vi "Check DataType with Cacher.vi"(0 "key":string, 2 "Type":T1) -> (4 "cacher":variant, 5 "match?":bool, 6 "stored type":T1, 7 "error out":errorcluster)   [LabVIEW 2017]
uses:
  <vilib>/Utility/Data Type/Type Definitions/Data Type.ctl
  <vilib>/Utility/Data Type/NI_Data Type.lvlib
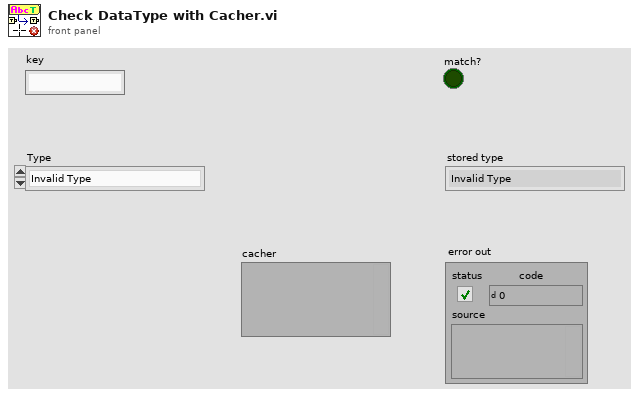
[diagram p1: front panel]
types:
  T1 = typedef "NI_Data Type.lvlib/Data Type.ctl" = enum8{"Invalid Type", "Void", "I8", "I16", "I32", "I64", "U8", "U16", "U32", "U64", "Single Float", "Double Float", "Extended Float", "Single Complex", "Double Complex", "Extended Complex", "Enum U8", "Enum U16", "Enum U32", "Enum U64", "Single Float With Unit", "Double Float With Unit", "Extended Float With Unit", "Single Complex with Unit", "Double Complex with Unit", "Extended Complex with Unit", "Boolean", "String", "Path", "Picture", "Tag", "Array", "Cluster", "Variant", "LV Variant", "Waveform", "Timestamp", "Digital Waveform", "Digital Data", "ExpressData", "Refnum", "External Data", "VI", "Poly VI", "LabVIEW Class Instance", "Fixed Point"}
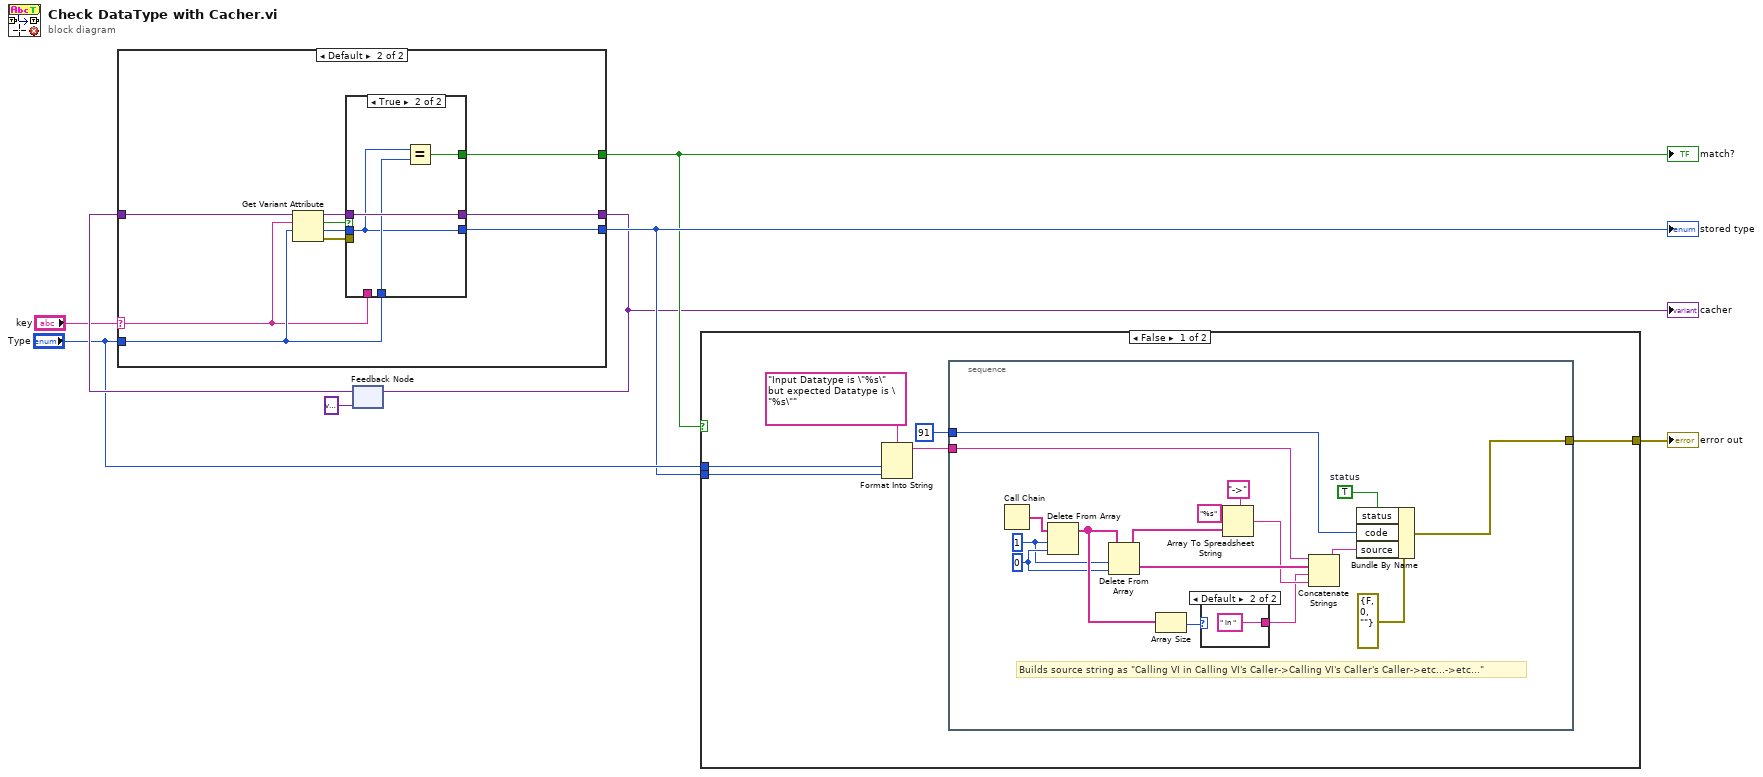
[diagram p0: block diagram]
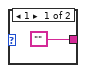
[diagram p2: hidden frame]
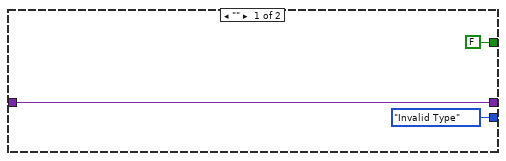
[diagram p4: hidden frame]
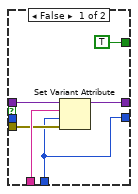
[diagram p5: hidden frame]
diagram:
  n1 = feedback #1(variant) -> (w7:variant)
  n2 = case shown="Default" "key" {
    selector: "key" -> [_ w16]
    tunnel: w7 -> [w11 w13]
    tunnel: [w11 w12] -> w1
    tunnel: "Type" -> [_ w17]
    tunnel: [FALSE w15] -> w2
    tunnel: [Data_Type."Invalid Type" ("Type") w14] -> w3
    frame "" {
    }
    frame Default {
      n3 = Get Variant Attribute(Variant=w13, name=w16, default value (empty Variant)=w17) -> (duplicate Variant=w21:variant, found=w20:bool, value=w19:T1, error out=w18:errorcluster)  [unwired: 1 in]
      n4 = case shown="True" w20 {
        tunnel: w21 -> [w27 w31]
        tunnel: w16 -> [w26 _]
        tunnel: w19 -> [_ w28]
        tunnel: w18 -> [w25 _]
        tunnel: [w24 w31] -> w12
        tunnel: w17 -> [w22 w30]
        tunnel: [TRUE w29] -> w15
        tunnel: [w22 w28] -> w14
        frame False {
          n5 = Set Variant Attribute(Variant=w27, name=w26, value=w22, error in=w25) -> (Variant out=w24:variant)  [unwired: 2 out]
        }
        frame True {
          n6 = Equal?(x=w28, y=w30) -> (x = y?=w29:bool)
        }
      }
    }
  }
  "cacher" <- w1
  "match?" <- w2
  "stored type" <- w3
  n7 = feedback-in #1(w1) -> ()
  n8 = case shown="False" w2 {
    tunnel: [w37 _] -> w5
    tunnel: "Type" -> [w33 _]
    tunnel: w3 -> [w32 _]
    frame False {
      n9 = Format Into String(format string="Input Datatype is \"%s\" but expected Datatype is \"%s\"", w33, w32) -> (resulting string=w34:string)  [unwired: 2 in, 1 out]
      n10 = stacked-sequence {
        tunnel: [w50] -> w37
        tunnel: w34 -> [w51]
        tunnel: 91 ("code") -> [w47]
        frame #0 {
          w44 = 0 ("Index")
          w43 = 1 ("Length")
          w48 = TRUE  # status
          # "Builds source string as \"Calling VI in Calling VI's Caller->Calling VI's Caller's Caller->etc...->etc...\""
          n11 = Call Chain() -> (call chain=w38:string[])
          n12 = Delete From Array(array=w38, length=w43, index=w44) -> (array with subset deleted=w54:string[])  [unwired: 1 out]
          n13 = Delete From Array(array=w54, length=w43, index=w44) -> (deleted portion=w53:string[], array with subset deleted=w45:string[])
          n14 = Array Size(array=w54) -> (size(s)=w52:i32)
          n15 = case shown="Default" w52 {
            tunnel: ["" " in " ("Format String")] -> w40
            frame 1 {
            }
            frame Default {
            }
          }
          n16 = Array To Spreadsheet String(delimiter (Tab)="->", array=w45, 3:"%s" ("format string")) -> (spreadsheet string=w41:string)
          n17 = Concatenate Strings(w51, w53, w40, w41) -> (w49:string)
          n18 = Bundle By Name(cluster=errorcluster {"status"=FALSE, "code"=0, "source"=""} ("error out"), "status"=w48, "code"=w47, "source"=w49) -> (w50:errorcluster)
        }
      }
    }
    frame True {
    }
  }
  "error out" <- w5
